vi "scan2d_generate_stage_positions.vi"(8 "error in (no error)":errorcluster, 10 "scan-settings":T1, 11 "scan_panel in":refnum<class "scan_2d.lvclass">) -> (0 "error out":errorcluster, 1 "y_positions":dbl[](array[numeric]), 2 "x_positions (mm)":dbl[](array[numeric]), 3 "scan_panel out":refnum<class "scan_2d.lvclass">)   [LabVIEW 2015, in "scan_2d.lvclass"]
uses:
  scan_2d.lvclass
  scan_2d_stage_settings.ctl
  scan_2d.lvclass/scan_2d.ctl
  <vilib>/Analysis/1siggen.llb/Ramp Pattern by Samples.vi
  <vilib>/Analysis/NI_AALBase.lvlib
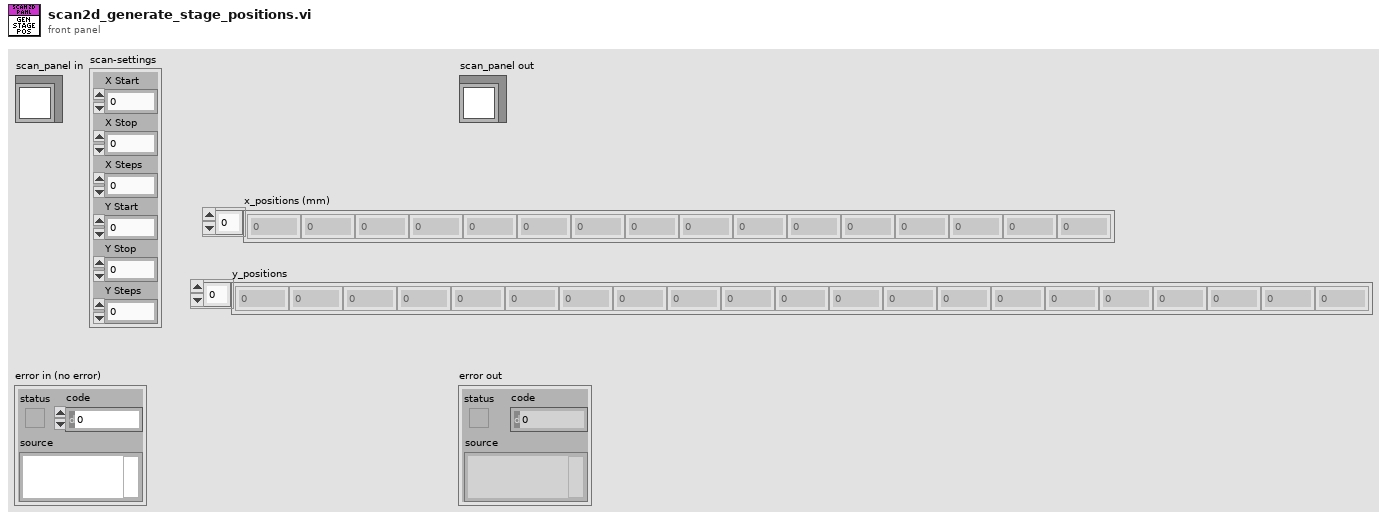
[diagram p1: front panel]
types:
  T1 = typedef "scan_2d_stage_settings.ctl" = cluster{"X Start":dbl, "X Stop":dbl, "X Steps":u32, "Y Start":dbl, "Y Stop":dbl, "Y Steps":u32}
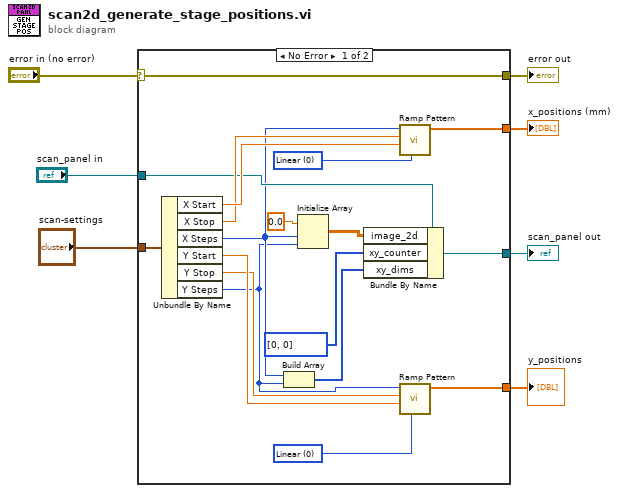
[diagram p0: block diagram]
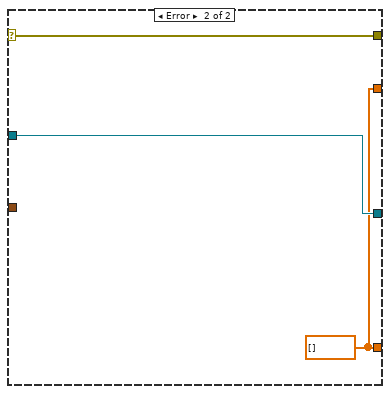
[diagram p2: hidden frame]
diagram:
  n1 = case shown="No Error" "error in (no error)" {
    selector: "error in (no error)" -> [w25 w28]
    tunnel: [w25 w28] -> w2
    tunnel: [w12 w27] -> w5
    tunnel: "scan_panel in" -> [w13 w27]
    tunnel: "scan-settings" -> [w24 _]
    tunnel: [w22 w26] -> w4
    tunnel: [w16 w26] -> w1
    frame No Error {
      w19 = u16 0 items=["Linear", "Logarithmic"] ("type")
      w23 = u16 0 items=["Linear", "Logarithmic"] ("type")
      n2 = Unbundle By Name(w24) -> ("X Start"=w21:dbl, "X Stop"=w20:dbl, "X Steps"=w10:u32, "Y Start"=w18:dbl, "Y Stop"=w17:dbl, "Y Steps"=w9:u32)
      n3 = Build Array(w10, w9) -> (w8:u32[])
      n4 = Initialize Array(0.0 ("element"), w10, w9) -> (w14:dbl[][])
      n5 = Bundle By Name(cluster=w13, "image_2d"=w14, "xy_counter"=u32[] [0, 0], "xy_dims"=w8) -> (w12:refnum<class "scan_2d.lvclass">)
      n6 = call-poly <vilib>:"Ramp Pattern.vi"("type"=w23, "start"=w21, "end"=w20, "samples"=w10) -> ("Ramp Pattern"=w22:dbl[])  [unwired: 6 in, 1 out]
      n7 = call-poly <vilib>:"Ramp Pattern.vi"("type"=w19, "start"=w18, "end"=w17, "samples"=w9) -> ("Ramp Pattern"=w16:dbl[])  [unwired: 6 in, 1 out]
    }
    frame Error {
      w26 = dbl[] [] ("Ramp Pattern")
    }
  }
  "error out" <- w2
  "scan_panel out" <- w5
  "x_positions (mm)" <- w4
  "y_positions" <- w1
